vi "Robo Team Send In action.vi"(8 "error in (no error)":errorcluster) -> (0 "error out":errorcluster)   [LabVIEW 2015]
uses:
  Robo Team Globals.vi
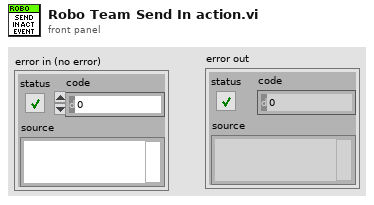
[diagram p1: front panel]
types:
  T1 = typedef "Robo System State Refs.ctl" = cluster{"Engage Motor":refnum<vi>, "Auto Level":refnum<vi>, "IMU led":refnum<vi>, "Evaluate Enable":refnum<vi>, "Motor Led":refnum<vi>, "Error Descript":refnum<vi>, "Error Led":refnum<vi>, "Error":refnum<vi>}
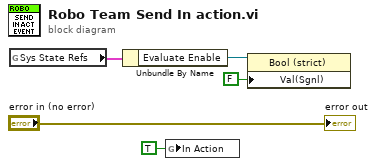
[diagram p0: block diagram]
diagram:
  n1 = global read "Robo Team Globals.vi" "Sys State Refs"() -> (w5:T1)
  n2 = Unbundle By Name(w5) -> ("Evaluate Enable"=w4:refnum<vi>)
  n3 = global write "Robo Team Globals.vi" "In Action"(TRUE ("In Action")) -> ()
  n4 = property class="Bool (strict)"(reference=w4, "Val(Sgnl)"=FALSE ("Value (Signaling)")) -> ()  [unwired: 1 in, 2 out]
  "error out" <- "error in (no error)"
